vi "Set Channel Name.vi"(8 "error in (no error)":errorcluster, 10 "Channel Name":string, 11 "Parameter in":refnum<class "Abstract Sensor Parameter.lvclass">) -> (0 "error out":errorcluster, 3 "Parameter out":refnum<class "Abstract Sensor Parameter.lvclass">)   [LabVIEW 2013, in "Parameter.lvlib" / "Abstract Sensor Parameter.lvclass"]
uses:
  Abstract Sensor Parameter.lvclass
  Abstract Sensor Parameter.lvclass/Abstract Sensor Parameter.ctl
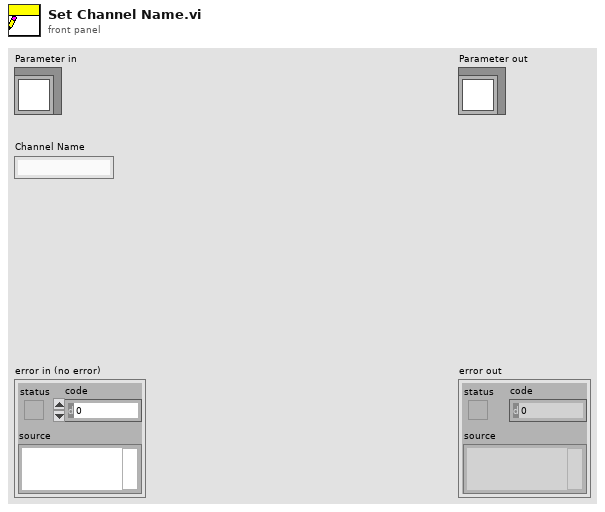
[diagram p1: front panel]
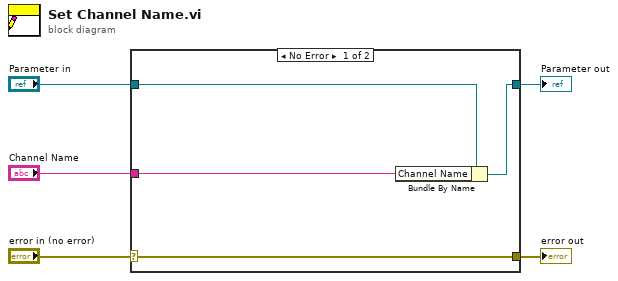
[diagram p0: block diagram]
diagram:
  n1 = case shown="No Error" "error in (no error)" {
    selector: "error in (no error)" -> [w9 w10]
    tunnel: [w9 w10] -> w4
    tunnel: [w7 w11] -> w2
    tunnel: "Parameter in" -> [w8 w11]
    tunnel: "Channel Name" -> [w6 _]
    frame No Error {
      n2 = Bundle By Name(cluster=w8, "Channel Name"=w6) -> (w7:refnum<class "Abstract Sensor Parameter.lvclass">)
    }
    frame Error {
    }
  }
  "error out" <- w4
  "Parameter out" <- w2
